vi "CircleCont.vi"(9 "ContPow":T5, 10 "NumSides":dbl, 11 "Diameter":dbl) -> (3 "PathSupreme":T1)   [LabVIEW 2014]
uses:
  TypeDefs/PowerSpeed.ctl
  TypeDefs/PathSupreme.ctl
  PSup2SCAN/Sub/VelocityProfile.ctl
  PSup2SCAN/Sub/PathCut.ctl
  PSup2SCAN/Sub/Segment.ctl
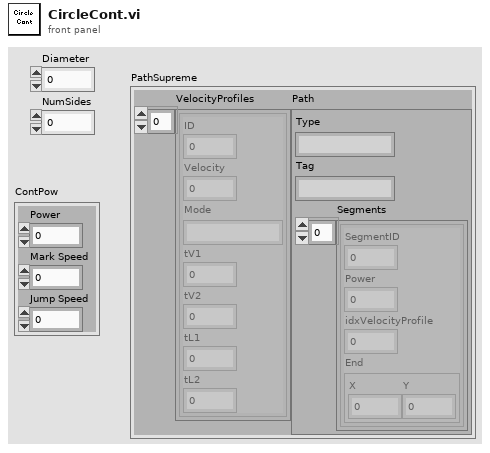
[diagram p1: front panel]
types:
  T1 = typedef "PathSupreme.ctl" = cluster{"VelocityProfiles":T2[], "Path":T3}
  T2 = typedef "VelocityProfile.ctl" = cluster{"ID":u32, "Velocity":dbl, "Mode":string, "tV1":u32, "tV2":u32, "tL1":u32, "tL2":u32}
  T3 = typedef "PathCut.ctl" = cluster{"Type":string, "Tag":string, "Segments":T4[]}
  T4 = typedef "Segment.ctl" = cluster{"SegmentID":u16, "Power":sgl, "idxVelocityProfile":u16, "End":cluster{"X":sgl, "Y":sgl}}
  T5 = typedef "PowerSpeed.ctl" = cluster{"Power":dbl, "Mark Speed":dbl, "Jump Speed":dbl}
  T6 = typedef "Point2DwSlope.ctl" = cluster{"X":sgl, "Y":sgl, "Slope":dbl}
  T7 = cluster{"VertexArray":T6[], "OnOffAr":enum16{"On", "Off"}[]}
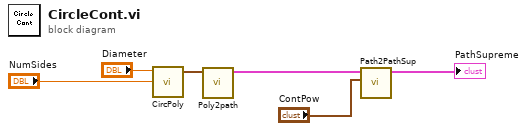
[diagram p0: block diagram]
diagram:
  n1 = call "CircPoly.vi"("NumSides"="NumSides", "Diameter"="Diameter") -> ("VertexArray"=w3:T6[])  [unwired: 9 in]
  n2 = call "Poly2path.vi"("VertexArray"=w3) -> ("Path"=w4:T7)  [unwired: 10 in]
  n3 = call "Path2PathSup.vi"("PowerSpeed"="ContPow", "Combined"=w4) -> ("PathSupreme"=→"PathSupreme":T1)  [unwired: 9 in]
